vi "Cryo-Con Set Manual Heater Value.vi"(8 "error in (no error)":errorcluster, 10 "Set heat %":dbl, 11 "VISA Resource Name":refnum<visa-resource-name>) -> (0 "error out":errorcluster, 2 "resulting string":string, 3 "VISA Resource Name Out":refnum<visa-resource-name>)   [LabVIEW 2019]
uses:
  GPIB/VISA  Send Receive.vi
panel:
  out "data string out":string
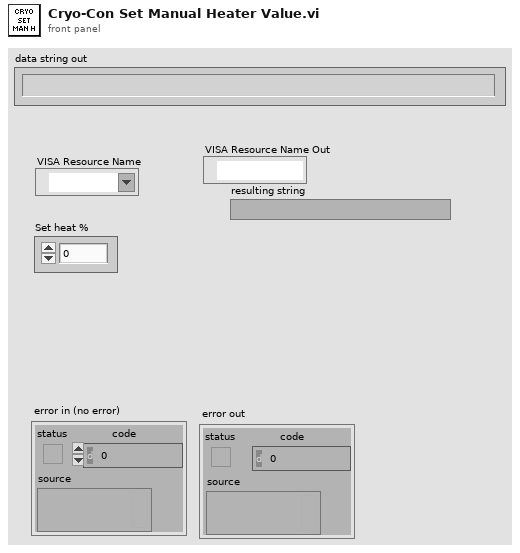
[diagram p1: front panel]
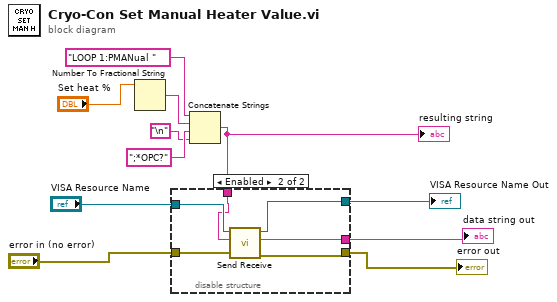
[diagram p0: block diagram]
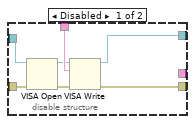
[diagram p2: hidden frame]
diagram:
  n1 = Number To Fractional String(number="Set heat %") -> (F-format string=w6:string)  [unwired: 3 in]
  n2 = Concatenate Strings("LOOP 1:PMANual " ("format string"), w6, ";*OPC?" ("string"), "\n") -> (w8:string)
  "resulting string" <- w8
  n3 = disable-structure shown="Enabled" {
    disable-tunnel: [w18 w21] -> w11
    disable-tunnel: [w17 w20] -> w10
    disable-tunnel: "error in (no error)" -> [w16 w24]
    disable-tunnel: w8 -> [w15 w22]
    disable-tunnel: "VISA Resource Name" -> [w12 w23]
    disable-tunnel: [_ w19] -> w1
    frame Disabled {
      n4 = VISA Open(error in (no error)=w16, VISA resource name=w12) -> (VISA resource name=w13:refnum<visa-resource-name>, error out=w14:errorcluster)  [unwired: 3 in]
      n5 = VISA Write(VISA resource name=w13, write buffer=w15, error in (no error)=w14) -> (VISA resource name out=w18:refnum<visa-resource-name>, error out=w17:errorcluster)  [unwired: 1 out]
    }
    frame Enabled {
      n6 = call-poly "Send Receive.vi"("error in (no error)"=w24, "data string in"=w22, "VISA Resource Name"=w23) -> ("error out"=w20:errorcluster, "data string out"=w19:string, "VISA Resource Name Out"=w21:refnum<visa-resource-name>)  [unwired: 6 in]
    }
  }
  "error out" <- w10
  "VISA Resource Name Out" <- w11
  "data string out" <- w1
